vi "QUEUE-REASON.vi"() -> ()   [LabVIEW 2013]
panel:
  in  "stop":bool
  out "Waveform Chart":dbl(graph)
  in  "SEND":bool
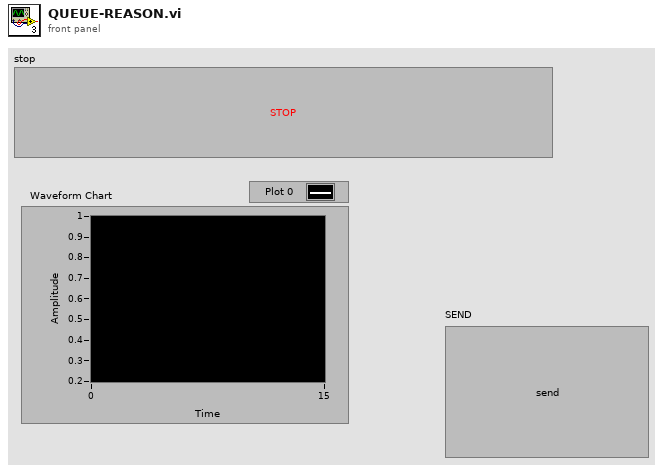
[diagram p1: front panel]
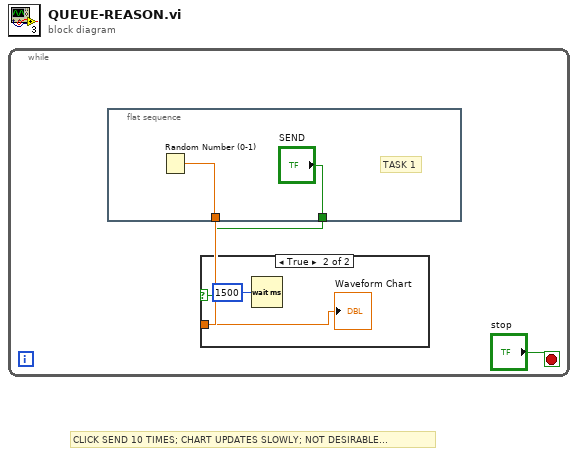
[diagram p0: block diagram]
diagram:
  # "CLICK SEND 10 TIMES; CHART UPDATES SLOWLY; NOT DESIRABLE..."
  n1 = while {
    stop <- "stop" stop-if-true
    n2 = flat-sequence {
      tunnel: [w7] -> w3
      tunnel: ["SEND"] -> w2
      frame #0 {
        # "TASK 1"
        n3 = Random Number (0-1)() -> (number: 0 to 1=w7:dbl)
      }
    }
    n4 = case shown="True" w2 {
      tunnel: w3 -> [_ w5]
      frame False {
      }
      frame True {
        n5 = Wait (ms)(milliseconds to wait=u32 1500) -> ()  [unwired: 1 out]
        "Waveform Chart" <- w5
      }
    }
  }
